vi "lfs_measure_black line.vi"(7 "ff":i32, 8 "error in (no error)":errorcluster, 9 "Position in":T1, 11 "limit":dbl) -> (0 "error out":errorcluster, 1 "Position  out":T1, 2 "0:R 1:L":bool[](array[boolean]), 3 "move cm":dbl, 4 "black?":bool)   [LabVIEW 2019]
uses:
  move/position cluster.ctl
  <vilib>/Platform/TimedLoop/XDataNode/timing_clust.ctl
  <vilib>/Platform/TimedLoop/XDataNode/nitl_modes.ctl
  <vilib>/Platform/TimedLoop/XDataNode/wakeup.ctl
  <vilib>/platform/TimedLoop/XDataNode/XDataNode.xnode
  <vilib>/Platform/TimedLoop/XDataNode/XDNodeRunTimeDep.lvlib
panel:
  out "Waveform Chart":T2(graph)
  out "process":dbl[](array[numeric])
  in  "stop":bool
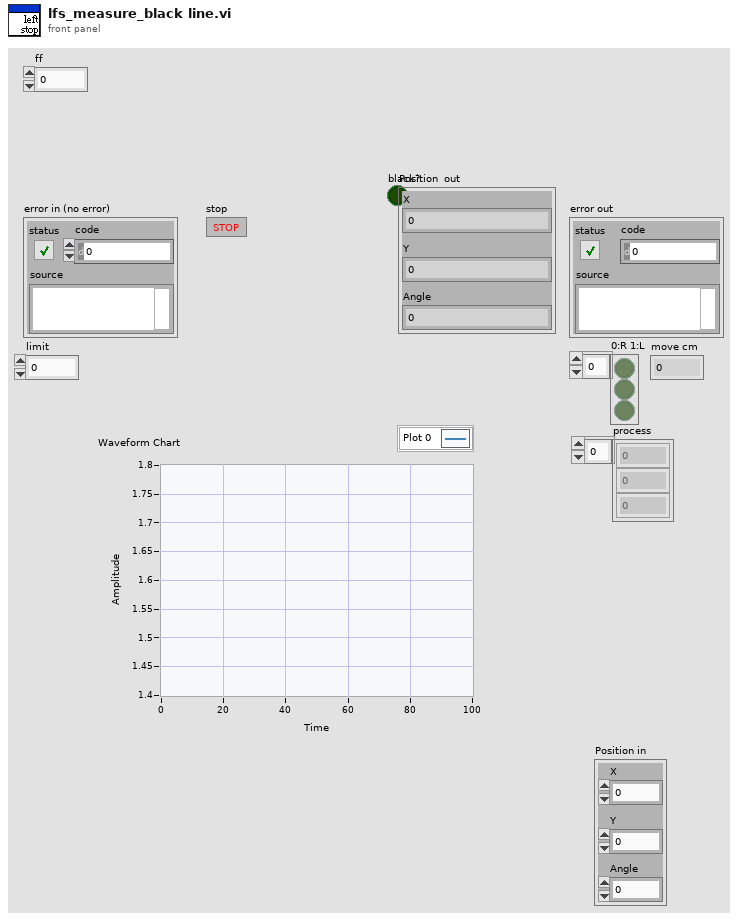
[diagram p1: front panel]
types:
  T1 = typedef "position cluster.ctl" = cluster{"X":dbl, "Y":dbl, "Angle":dbl}
  T2 = cluster{"dbl Scaled Value left":dbl, "dbl Scaled Value right":dbl}
  T3 = typedef "XDNodeRunTimeDep.lvlib/timing_clust.ctl" = cluster{"Expected End [f-1]":u64, "Actual End [f-1]":u64, "Finished Late? [f-1]":bool, "Expected End [i-1]":u64, "Actual End [i-1]":u64, "Finished Late? [i-1]":bool, "Expected Start [i]":u64, "Actual Start [i]":u64, "Expected Start [f]":u64, "Actual Start [f]":u64, "Source Name":string, "Structure Name":string, "Period":i64, "Deadline":i64, "Offset":i64, "Start":i64, "Priority":i32, "Timeout":i32, "Mode":T4, "Wakeup Reason":T5, "Error":errorcluster, "Source Type":string, "Secondary Source Type":string, "Global End Time":u64, "Global Start Time":u64, "Frame Duration":u64, "Iteration Duration":u64, "Assigned CPU":i32, "I/O Scan Engine Mode":u32}
  T4 = typedef "XDNodeRunTimeDep.lvlib/nitl_modes.ctl" = enum32{"No Change", "Process missed periods, maintain original phase", "Discard missed periods, maintain original phase", "Process missed periods, ignore original phase", "Discard missed periods, ignore original phase"}
  T5 = typedef "XDNodeRunTimeDep.lvlib/wakeup.ctl" = enum32{"Normal", "Aborted", "Asynchronous wakeup", "Timing source error", "Timed loop error", "Timeout"}
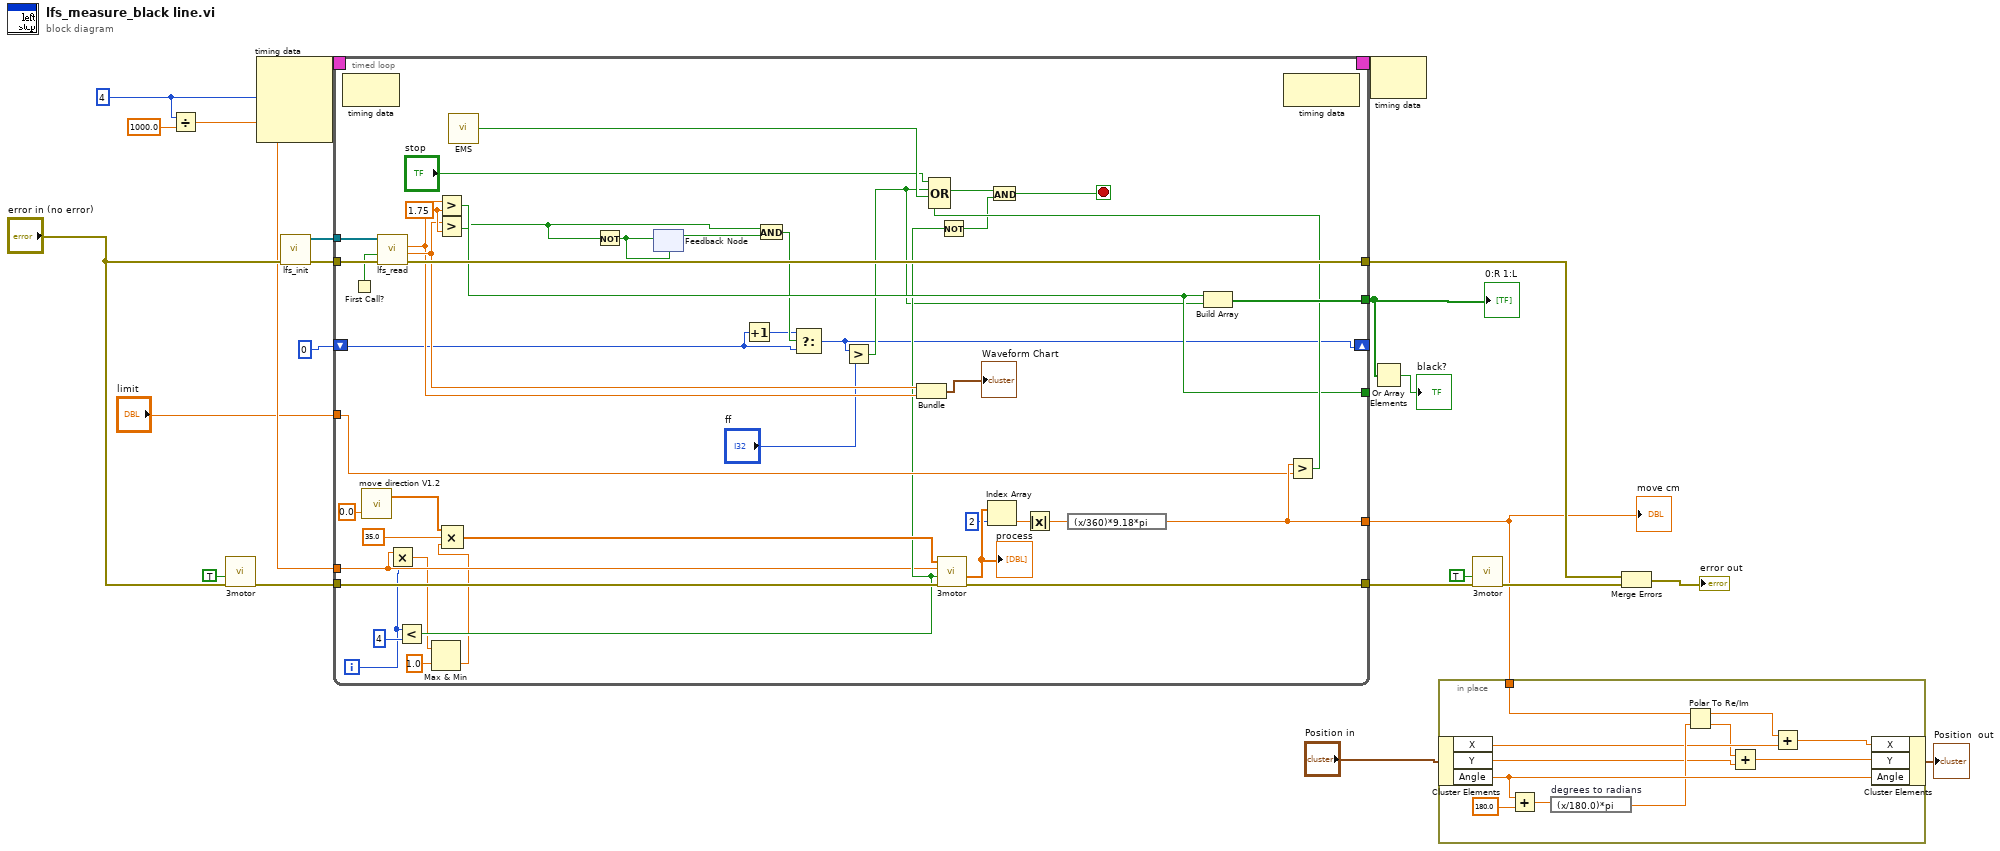
[diagram p0: block diagram]
diagram:
  w12 = i64 4 ("Period")
  n1 = Divide(x=w12, y=1000.0) -> (x/y=w10:dbl)
  n2 = call "3motor.vi"("error in (no error)"="error in (no error)", "Reset"=TRUE) -> ("error out"=w15:errorcluster)  [unwired: 8 in, 1 out]
  n3 = node-c288(w12) -> (w22:T3)  [unwired: 3 in]
  n4 = call "lfs_init.vi"("error in (no error)"="error in (no error)") -> ("error out"=w20:errorcluster, "lfs ref"=w19:refnum<class "IR sensor.lvclass">[])  [unwired: 9 in]
  n5 = timed-loop {
    timing: w22 -> [_]
    timing-out: [_] -> w21
    tunnel: w20 -> [w66]
    tunnel: w19 -> [w65]
    tunnel: [w64] -> w18
    tunnel: [w61] -> w17
    tunnel: w15 -> [w60]
    tunnel: w10 -> [w38]
    tunnel: [w52] -> w2
    tunnel: [w50] -> w5
    tunnel: "limit" -> [w49]
    tunnel: [w44] -> _
    shift-right: [w23] -> _
    shift-left: 0 -> [w26]
    i -> [w37]
    stop <- w39 stop-if-true
    w63 = 1.75
    n6 = node-c288() -> ()  [unwired: 1 in, 1 out]
    n7 = First Call?() -> (First Call?: T/F=w33:bool)
    n8 = call "move direction V1.2.vi"("theta"=0.0) -> ("out array"=w58:dbl[])  [unwired: 1 in, 1 out]
    n9 = call "lfs_read.vi"("error in (no error)"=w66, "initialize"=w33, "lfs ref in"=w65) -> ("error out"=w64:errorcluster, "dbl Scaled Value left"=w47:dbl, "dbl Scaled Value right"=w46:dbl)  [unwired: 5 in, 1 out]
    n10 = Multiply(x=w38, y=w37) -> (x*y=w36:dbl)
    n11 = Less?(x=w37, y=4) -> (x < y?=w42:bool)
    n12 = Max & Min(x=w36, y=1.0) -> (min(x,y)=w34:dbl)  [unwired: 1 out]
    n13 = Greater?(x=w46, y=w63) -> (0:w44:bool)
    n14 = Greater?(x=w47, y=w63) -> (0:w30:bool)
    n15 = Compound Arithmetic op=MULTIPLY(w58, 35.0 ("y"), w34) -> (w56:dbl[])
    n16 = call "EMS.vi"() -> ("A/DIO4 (Pin 19)"=w62:bool)
    n17 = Not(x=w30) -> (.not. x?=w29:bool)
    n18 = feedback-in #1(w29) -> ()
    n19 = feedback #1(w29) -> (w31:bool)
    n20 = Increment(x=w26) -> (x+1=w27:i32)
    n21 = And(x=w30, y=w31) -> (x .and. y?=w28:bool)
    n22 = Select(t=w27, s=w28, f=w26) -> (s? t:f=w23:i32)
    n23 = Greater?(x=w23, y="ff") -> (0:w25:bool)
    n24 = Bundle("dbl Scaled Value left"=w47, "dbl Scaled Value right"=w46) -> (→"Waveform Chart":T2)  [unwired: 1 in]
    n25 = call "3motor.vi"("error in (no error)"=w60, "Reset"=w42, "dt(s)"=w38, "Motor speed"=w56) -> ("error out"=w61:errorcluster, "encoder array"=w55:dbl[])  [unwired: 6 in]
    "process" <- w55
    n26 = Not(x=w42) -> (.not. x?=w40:bool)
    n27 = Index Array(array=w55, index=2) -> (element=w53:dbl)
    n28 = Absolute Value(x=w53) -> (abs(x)=w51:dbl)
    n29 = expression code="(x/360)*9.18*pi" ("RPM to radian/s")(w51) -> (w50:dbl)
    n30 = Build Array(w44, w25) -> (w52:bool[])
    n31 = node-c288() -> ()  [unwired: 1 in, 1 out]
    n32 = Greater?(x=w50, y=w49) -> (0:w48:bool)
    n33 = Compound Arithmetic op=OR("stop", w25, w62, w48) -> (w41:bool)
    n34 = And(x=w41, y=w40) -> (x .and. y?=w39:bool)
  }
  "0:R 1:L" <- w2
  "move cm" <- w5
  n35 = node-c288(w21) -> ()  [unwired: 1 out]
  n36 = Or Array Elements(Boolean array=w2) -> (logical OR=→"black?":bool)
  n37 = in-place {
    in-place-border: w5 -> [w75]
    n38 = in-place-cluster #2("Position in") -> ("X"=w73:dbl, "Y"=w71:dbl, "Angle"=w79:dbl)
    n39 = Add(x=w79, y=180.0) -> (x+y=w77:dbl)
    n40 = expression code="(x/180.0)*pi" "degrees to radians"(w77) -> (w76:dbl)
    n41 = Polar To Re/Im(2:w76, 3:w75) -> (0:w72:dbl, 1:w74:dbl)
    n42 = Add(x=w72, y=w71) -> (x+y=w70:dbl)
    n43 = Add(x=w74, y=w73) -> (x+y=w69:dbl)
    n44 = in-place-cluster #2("X"=w69, "Y"=w70, "Angle"=w79) -> (→"Position  out":T1)
  }
  n45 = call "3motor.vi"("error in (no error)"=w17, "Reset"=TRUE) -> ("error out"=w9:errorcluster)  [unwired: 8 in, 1 out]
  n46 = Merge Errors(w18, w9) -> (→"error out":errorcluster)
